vi "CalcWidthSave.vi"() -> ()   [LabVIEW 2017]
uses:
  <vilib>/Analysis/baseanly.llb/Mean (DBL).vi
  <vilib>/Analysis/NI_AALBase.lvlib
panel:
  in  "Folder Path":path
  in  "Pixel size, um":dbl
  in  "Focus, mm":dbl
  in  "Rotate, deg":dbl=1.6 format="%#_13g"
  in  "Threshold, %":dbl=2.0 format="%#_13g"
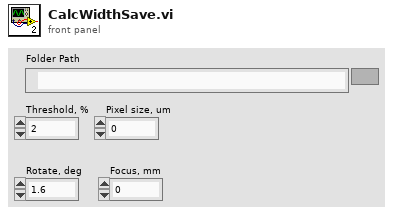
[diagram p1: front panel]
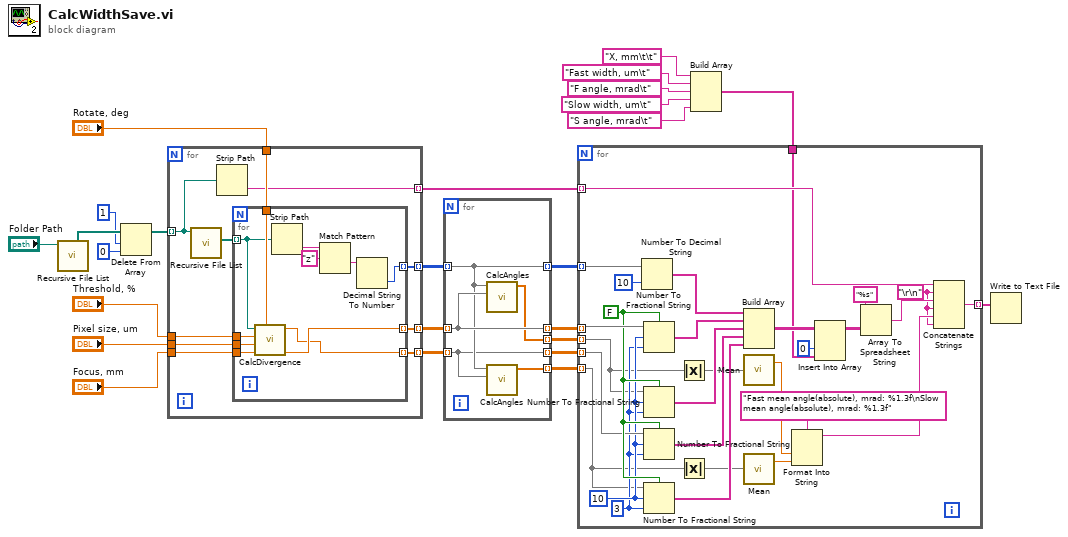
[diagram p0: block diagram]
diagram:
  n1 = call <vilib>:"Recursive File List.vi"("Folder Path"="Folder Path") -> ("All Folders"=w18:path[])  [unwired: 6 in, 4 out]
  n2 = Delete From Array(array=w18, length=1, index=0) -> (array with subset deleted=w15:path[])  [unwired: 1 out]
  n3 = for {
    tunnel: "Rotate, deg" -> [w35]
    tunnel: "Threshold, %" -> [w34]
    tunnel: "Pixel size, um" -> [w33]
    tunnel: "Focus, mm" -> [w32]
    tunnel: w15 -> [w30] mode=indexing
    tunnel: [w29] -> w20 mode=indexing
    tunnel: [w28] -> w10 mode=indexing
    tunnel: [w27] -> w9 mode=indexing
    tunnel: [w26] -> w11 mode=indexing
    n4 = call <vilib>:"Recursive File List.vi"("Folder Path"=w30) -> ("All Files in Dir"=w31:path[])  [unwired: 6 in, 4 out]
    n5 = Strip Path(path=w30) -> (name=w29:string)  [unwired: 1 out]
    n6 = for {
      tunnel: w35 -> [w46]
      tunnel: w34 -> [w45]
      tunnel: w33 -> [w44]
      tunnel: w32 -> [w43]
      tunnel: [w36] -> w27 mode=indexing
      tunnel: [w37] -> w28 mode=indexing
      tunnel: w31 -> [w42] mode=indexing
      tunnel: [w38] -> w26 mode=indexing
      n7 = call "CalcDivergence.vi"("Rotate, deg"=w46, "Focus, mm"=w43, "Pixel size, um"=w44, "Threshold, %"=w45, "path to PNG file"=w42) -> ("F Width, um"=w37:dbl, "S Width, um"=w36:dbl)  [unwired: 3 in, 2 out]
      n8 = Strip Path(path=w42) -> (name=w41:string)  [unwired: 1 out]
      n9 = Match Pattern(string=w41, regular expression="z") -> (after substring=w39:string)  [unwired: 1 in, 3 out]
      n10 = Decimal String To Number(string=w39) -> (number=w38:i32)  [unwired: 2 in, 1 out]
    }
  }
  n11 = for {
    tunnel: w11 -> [w50] mode=indexing
    tunnel: w10 -> [w51] mode=indexing
    tunnel: w9 -> [w49] mode=indexing
    tunnel: [w51] -> w8 mode=indexing
    tunnel: [w50] -> w7 mode=indexing
    tunnel: [w49] -> w6 mode=indexing
    tunnel: [w48] -> w5 mode=indexing
    tunnel: [w47] -> w4 mode=indexing
    n12 = call "CalcAngles.vi"("Widths, um"=w51, "Distances, mm"=w50) -> ("Angles, mrad"=w48:dbl[])  [unwired: 9 in]
    n13 = call "CalcAngles.vi"("Widths, um"=w49, "Distances, mm"=w50) -> ("Angles, mrad"=w47:dbl[])  [unwired: 9 in]
  }
  n14 = Build Array("X, mm\t\t" ("format string"), "Fast width, um\t" ("format string"), "F angle, mrad\t" ("format string"), "Slow width, um\t" ("format string"), "S angle, mrad\t" ("format string")) -> (w12:string[])
  n15 = for {
    tunnel: w20 -> [w79] mode=indexing
    tunnel: w8 -> [w74] mode=indexing
    tunnel: w6 -> [w65] mode=indexing
    tunnel: [w77] -> w19 mode=indexing
    tunnel: w7 -> [w76] mode=indexing
    tunnel: w12 -> [w71]
    tunnel: w5 -> [w53] mode=indexing
    tunnel: w4 -> [w54] mode=indexing
    w66 = FALSE ("use system decimal point (T)")
    w63 = i16 3 ("precision (6)")
    w64 = i16 10 ("width (-)")
    w56 = "\r\n"
    n16 = Number To Decimal String(number=w76, width (-)=i16 10) -> (decimal integer string=w75:string[])
    n17 = Number To Fractional String(use system decimal point (T)=w66, number=w74, width (-)=w64, precision (6)=w63) -> (F-format string=w73:string[])
    n18 = Number To Fractional String(use system decimal point (T)=w66, number=w53, width (-)=w64, precision (6)=w63) -> (F-format string=w67:string[])
    n19 = Number To Fractional String(use system decimal point (T)=w66, number=w65, width (-)=w64, precision (6)=w63) -> (F-format string=w62:string[])
    n20 = Number To Fractional String(use system decimal point (T)=w66, number=w54, width (-)=w64, precision (6)=w63) -> (F-format string=w61:string[])
    n21 = Absolute Value(x=w53) -> (abs(x)=w52:dbl[])
    n22 = Absolute Value(x=w54) -> (abs(x)=w55:dbl[])
    n23 = Build Array(w75, w73, w67, w62, w61) -> (w72:string[][])
    n24 = call-poly <vilib>:"Mean.vi"("X"=w52) -> ("mean"=w60:dbl)  [unwired: 1 out]
    n25 = call-poly <vilib>:"Mean.vi"("X"=w55) -> ("mean"=w59:dbl)  [unwired: 1 out]
    n26 = Format Into String(format string="Fast mean angle(absolute), mrad: %1.3f\nSlow mean angle(absolute), mrad: %1.3f", w60, w59) -> (resulting string=w57:string)  [unwired: 2 in, 1 out]
    n27 = Insert Into Array(array=w72, index (col)=0 ("index (row)"), new element=w71) -> (w70:string[][])  [unwired: 1 in]
    n28 = Array To Spreadsheet String(array=w70, 3:"%s" ("format string")) -> (spreadsheet string=w78:string)  [unwired: 1 in]
    n29 = Concatenate Strings(w79, w56, w78, w56, w57, w56) -> (w77:string)
  }
  n30 = Write to Text File(text=w19) -> ()  [unwired: 3 in, 3 out]
